vi "Get Output Voltage.vi"(8 "error in (no error)":errorcluster, 10 "Step index":i32, 11 "Ramp Use Case in":refnum<class "Ramp Voltage.lvclass">) -> (0 "error out":errorcluster, 2 "Output Voltage [V]":dbl, 3 "Ramp Use Case in 2":refnum<class "Ramp Voltage.lvclass">)   [LabVIEW 2020, in "High Level PSU With Tests.lvlib" / "Ramp Voltage.lvclass"]
uses:
  Ramp Voltage.lvclass
  Ramp Voltage.lvclass/Ramp Voltage.ctl
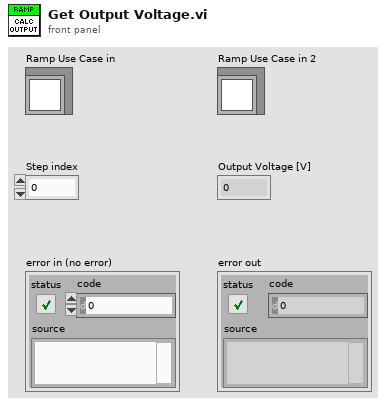
[diagram p1: front panel]
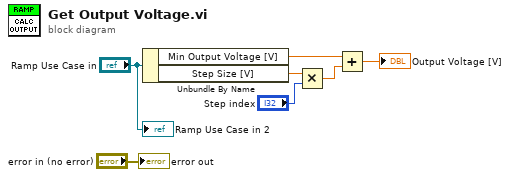
[diagram p0: block diagram]
diagram:
  n1 = Unbundle By Name("Ramp Use Case in") -> ("Min Output Voltage [V]"=w6:dbl, "Step Size [V]"=w7:dbl)
  n2 = Multiply(x=w7, y="Step index") -> (x*y=w2:dbl)
  n3 = Add(x=w6, y=w2) -> (x+y=→"Output Voltage [V]":dbl)
  "error out" <- "error in (no error)"
  "Ramp Use Case in 2" <- "Ramp Use Case in"
